vi "read station adcs port config.vi"(9 "ldf file name":string="CD701_CEM_LIN3_20230222", 10 "byte config file path":path, 11 "port":string="CD701_CEM_LIN3_20230222") -> (3 "ADCS LIN":T1={"Port"="LIN1", "HW select"=0, "XNET Cluster"="NIXNET_exampleLDF", "ByteCmd Path"=path "C:/Labview Code/System/ByteCmdConfig.txt"} {"HW select" items=["NI-XNET", "NI-CAN"]})   [LabVIEW 2018]
uses:
  <vilib>/CMC.AME/Inalfa ADCS/Ctl'Def/ADCS_LIN info.ctl
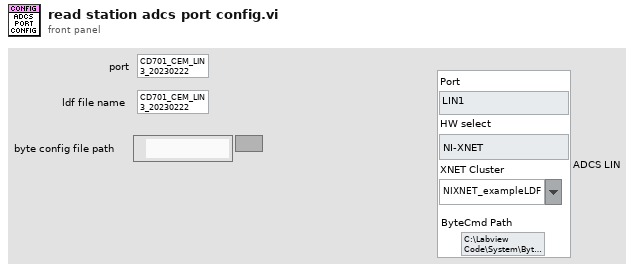
[diagram p1: front panel]
types:
  T1 = typedef "ADCS_LIN info.ctl" = cluster{"Port":string, "HW select":u16, "XNET Cluster":string, "ByteCmd Path":path}
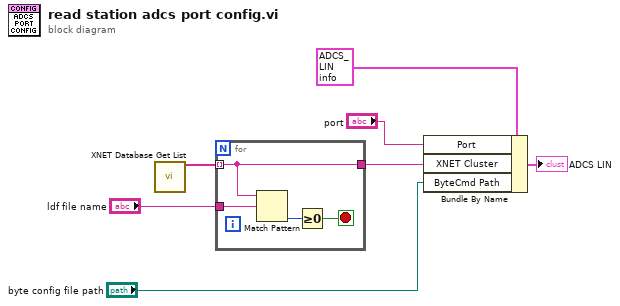
[diagram p0: block diagram]
diagram:
  n1 = call <vilib>:"XNET Database Get List.vi"() -> ("array of alias"=w7:string[])  [unwired: 13 in, 2 out]
  n2 = for {
    tunnel: w7 -> [w11] mode=indexing
    tunnel: [w11] -> w4
    tunnel: "ldf file name" -> [w10]
    stop <- w8 stop-if-true
    n3 = Match Pattern(string=w11, regular expression=w10) -> (offset past match=w9:i32)  [unwired: 1 in, 3 out]
    n4 = Greater Or Equal To 0?(x=w9) -> (x >= 0?=w8:bool)
  }
  n5 = Bundle By Name(cluster=T1 {"Port"="LIN1", "HW select"=0, "XNET Cluster"="NIXNET_exampleLDF", "ByteCmd Path"=path "C:/Labview Code/System/ByteCmdConfig.txt"} ("ADCS_LIN info"), "Port"="port", "XNET Cluster"=w4, "ByteCmd Path"="byte config file path") -> (→"ADCS LIN":T1)
